vi "API ID.vi"(11 "VolatusAPI in":refnum<class "VolatusAPI.lvclass">) -> (2 "ID":string)   [LabVIEW 2020, in "Volatus.lvlib" / "VolatusAPI.lvclass"]
uses:
  VolatusAPI.lvclass
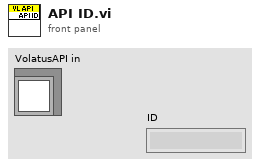
[diagram p1: front panel]
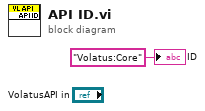
[diagram p0: block diagram]
diagram:
  "ID" <- "Volatus:Core" ("ID")
